vi "Init.vi"(8 "error in (no error)":errorcluster, 10 "Route":bool[][](array[boolean]), 11 "Channels":T1[](array[typedef])) -> (0 "error out":errorcluster, 3 "AudioSummaryValue out":refnum<class "AudioSummaryValue.lvclass">)   [LabVIEW 2022 SP3, in "VMR Server.lvlib" / "AudioSummaryValue.lvclass"]
uses:
  AudioSummaryValue.lvclass
  AudioSummaryValue.lvclass/AudioSummaryValue.ctl
  VMR Server Shared/Channel.ctl
  VMR Server Shared/VMR Server Shared.lvlib
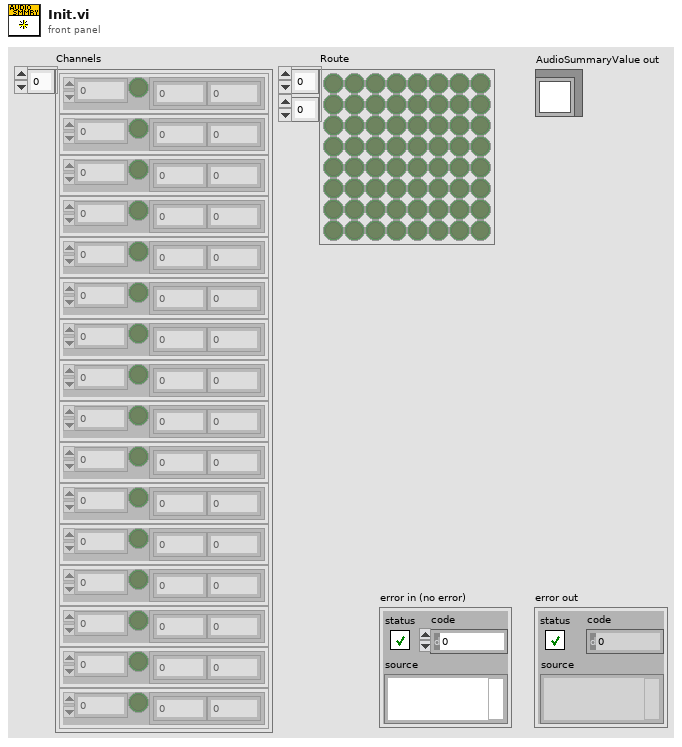
[diagram p1: front panel]
types:
  T1 = typedef "VMR Server Shared.lvlib/Channel.ctl" = cluster{"Gain":dbl, "Muted":bool, "Levels":cluster{"L":dbl, "R":dbl}}
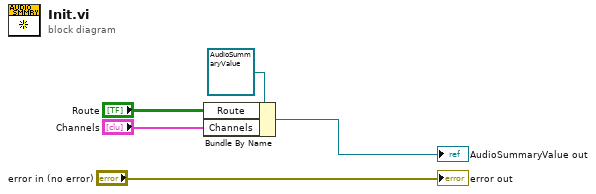
[diagram p0: block diagram]
diagram:
  n1 = Bundle By Name(cluster=refnum<class "AudioSummaryValue.lvclass"> refnum ("AudioSummaryValue in"), "Route"="Route", "Channels"="Channels") -> (→"AudioSummaryValue out":refnum<class "AudioSummaryValue.lvclass">)
  "error out" <- "error in (no error)"
